vi "Slave Select.vi"(7 "Slave Address":i32=-1 min=-1 max=30 step=1, 8 "error":errorcluster, 11 "VISA":refnum<visa-resource-name>) -> (0 "error out":errorcluster, 3 "VISA out":refnum<visa-resource-name>)   [LabVIEW 2023, in "TDK-Lambda GEN LAN Series.lvlib"]
doc: "This VI performs the addressing of any RS-485 slave units connected to the master unit. If the \"Slave Addr\" control is wired and it's value has changed since the last call, this VI sends \"INST:SEL nn\" to activate the new slave address.\n\nThis driver is called by each of higher-level drivers, so normally it is not used seperately in a LabView program.\n\nIf a slave at address \"nn\" is not detected, an error is returned on the \"error out\" string."
uses:
  TDK-Lambda GEN LAN Series.lvlib
panel:
  in  "Last Slave Address":i8=99
  out "error out 2":errorcluster
  # "Send Slave Address"
  # "TDK-Lambda Genesys \n LAN\n  DC Power Supplies"
  # "If \"Slave Address\" is wired \nand has changed,\nsend \"INSTRUMENT:SELECT\""
  # "( -1 = Default \n       = No Addr Change)"
  # "( info only)"
  # "(c) 2019 TDK-Lambda.  ALL RIGHTS RESERVED."
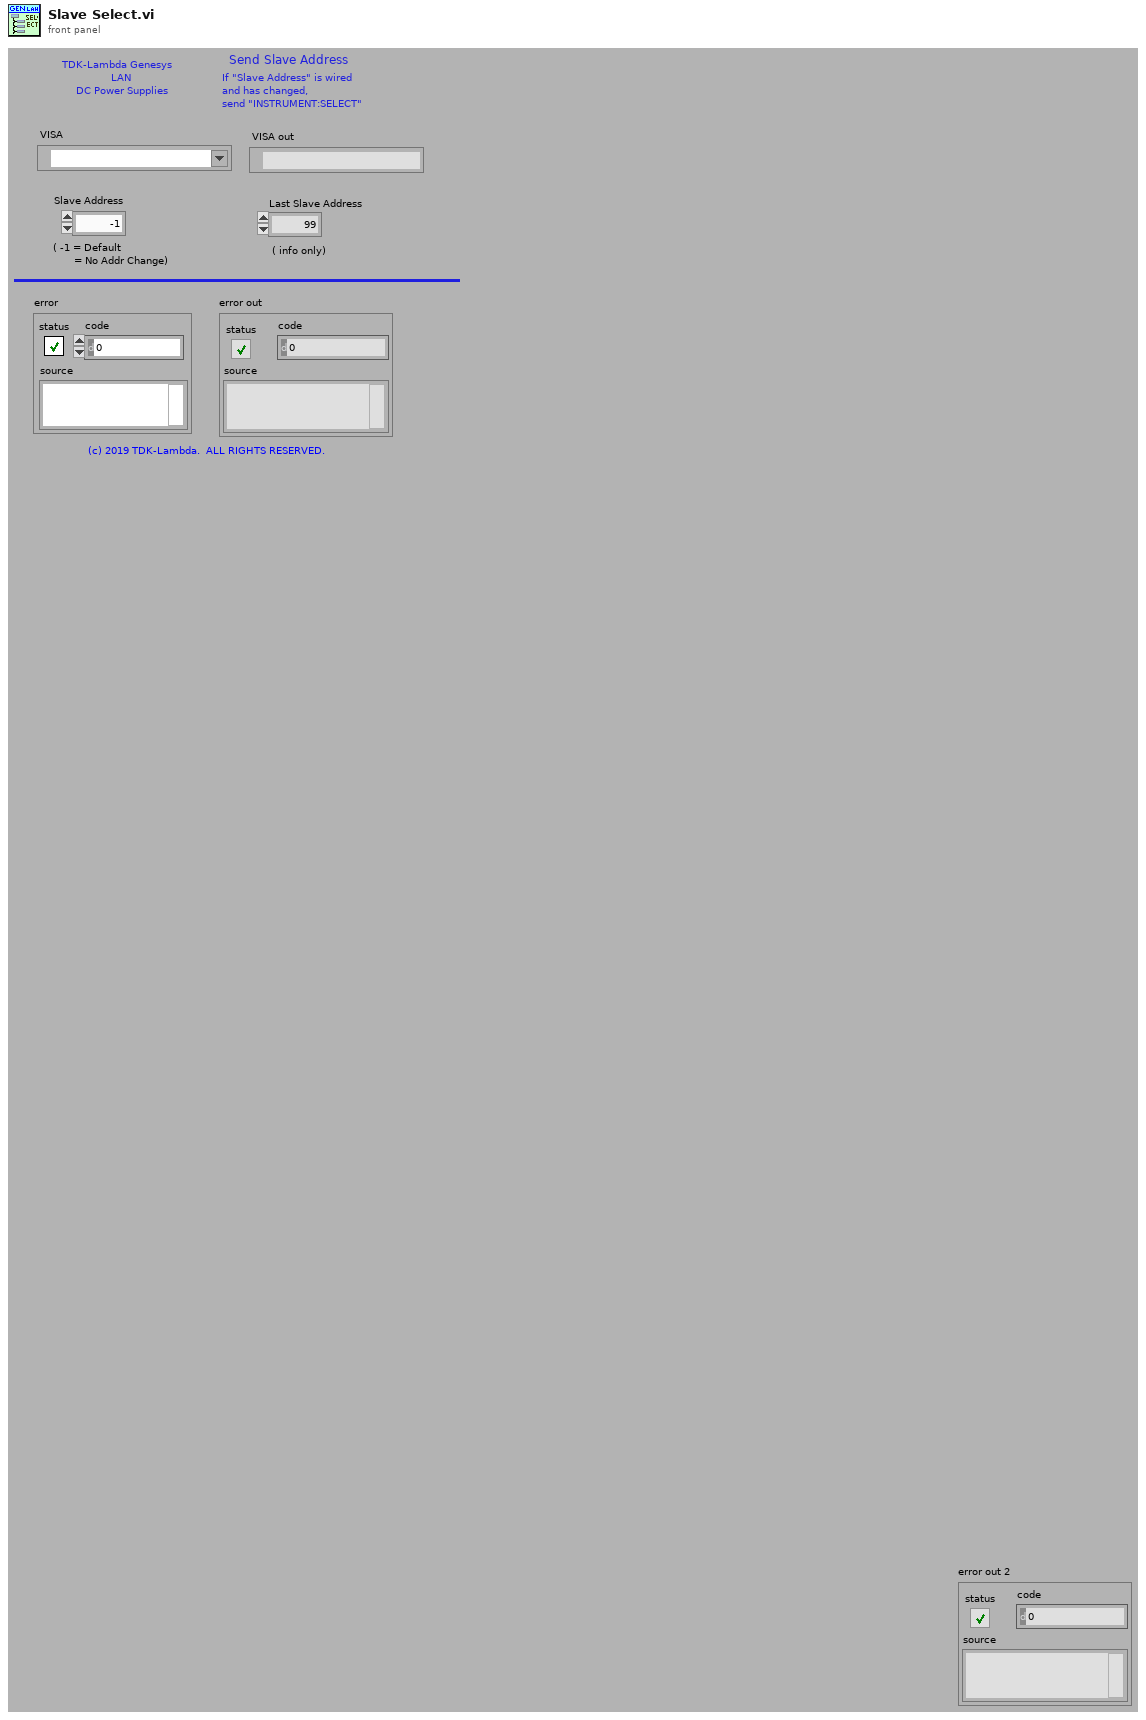
[diagram p1: front panel]
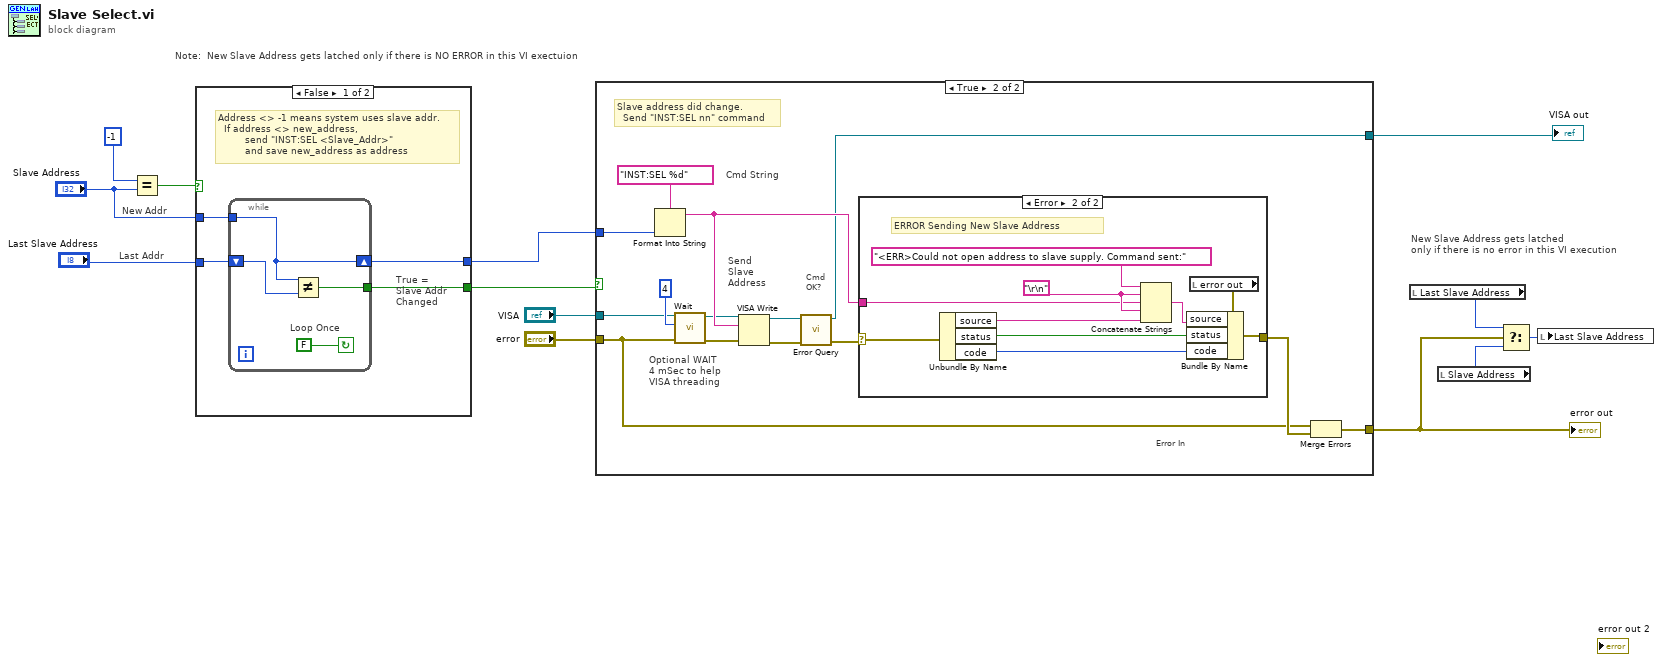
[diagram p0: block diagram]
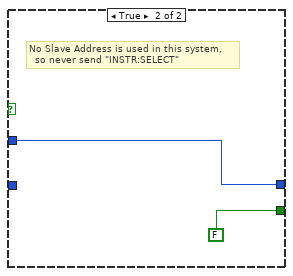
[diagram p4: hidden frame]
diagram:
  # "New Slave Address gets latched \nonly if there is no error in this VI execution"
  # "Note:  New Slave Address gets latched only if there is NO ERROR in this VI exectuion"
  # "Last Addr"
  # "New Addr"
  n1 = Equal?(x=i8 -1 ("y"), y="Slave Address") -> (x = y?=w13:bool)
  n2 = case shown="False" w13 {
    tunnel: "Slave Address" -> [w17 w22]
    tunnel: "Last Slave Address" -> [w16 _]
    tunnel: [w15 FALSE] -> w6
    tunnel: [w14 w22] -> w10
    frame False {
      # "True = \nSlave Addr \nChanged"
      # "Address <> -1 means system uses slave addr.  \n  If address <> new_address, \n         send \"INST:SEL <Slave_Addr>\"  \n         and save new_address as address"
      n3 = while {
        shift-right: [w18] -> w14
        shift-left: w16 -> [w20]
        tunnel: w17 -> [w18]
        tunnel: [w19] -> w15
        stop <- FALSE continue-if-true
        # "Loop Once"
        n4 = Not Equal?(x=w18, y=w20) -> (x != y?=w19:bool)
      }
    }
    frame True {
      # "No Slave Address is used in this system, \n  so never send \"INSTR:SELECT\""
    }
  }
  n5 = case shown="True" w6 {
    tunnel: [w24 w35] -> w5
    tunnel: w10 -> [_ w37]
    tunnel: [w25 w33] -> w9
    tunnel: "VISA" -> [w25 w26]
    tunnel: "error" -> [w24 w27]
    frame False {
      # "Slave address did not change.  \n  Do Not send \"INST:SEL\" command"
    }
    frame True {
      # "Optional WAIT \n4 mSec to help VISA threading"
      # "Error In"
      # "Slave address did change.  \n  Send \"INST:SEL nn\" command"
      # "Cmd String"
      # "Send \nSlave \nAddress"
      # "Cmd\nOK?"
      n6 = Format Into String(format string="INST:SEL %d", w37) -> (resulting string=w38:string)  [unwired: 2 in, 1 out]
      n7 = call "Wait.vi"("error"=w27, "Delay (20 mS)"=u32 4, "VISA"=w26) -> ("error out"=w30:errorcluster, "VISA out"=w31:refnum<visa-resource-name>)  [unwired: 7 in]
      n8 = VISA Write(VISA resource name=w31, write buffer=w38, error in (no error)=w30) -> (VISA resource name out=w29:refnum<visa-resource-name>, error out=w28:errorcluster)  [unwired: 1 out]
      n9 = call "Error Query.vi"("error"=w28, "VISA"=w29) -> ("error out"=w34:errorcluster, "VISA out"=w33:refnum<visa-resource-name>)  [unwired: 6 in, 2 out]
      n10 = case shown="Error" w34 {
        selector: w34 -> [w40 w44]
        tunnel: w38 -> [_ w46]
        tunnel: [w40 w45] -> w36
        frame No Error {
          # "New Slave Addressed Correctly.  \n  Sent \"INST:SEL <new addr>\" without error"
        }
        frame Error {
          w47 = "\r\n"
          # "ERROR Sending New Slave Address"
          n11 = Unbundle By Name(w44) -> ("source"=w43:string, "status"=w42:bool, "code"=w41:i32)
          n12 = Concatenate Strings("<ERR>Could not open address to slave supply. Command sent:" ("Source"), w47, w46, w47, w43) -> (w49:string)
          n13 = local read "error out"() -> (w50:errorcluster)
          n14 = Bundle By Name(cluster=w50, "source"=w49, "status"=w42, "code"=w41) -> (w45:errorcluster)
        }
      }
      n15 = Merge Errors(w27, w36) -> (w35:errorcluster)
    }
  }
  "error out" <- w5
  "VISA out" <- w9
  n16 = local read "Last Slave Address"() -> (w3:i8)
  n17 = local read "Slave Address"() -> (w2:i32)
  n18 = Select(t=w3, s=w5, f=w2) -> (s? t:f=w4:i32)
  n19 = local write "Last Slave Address"(w4) -> ()
